vi "Read FP Control.vi"(6 "Field name":string, 8 "error in (no error)":errorcluster, 10 "Control Name":string="Configuration", 11 "Measure Object in":refnum<class "Template Module.lvclass">) -> (0 "error out":errorcluster, 1 "Present":bool, 2 "Control Value":variant, 3 "Measure Object out":refnum<class "Template Module.lvclass">)   [LabVIEW 2018, in "Template Module.lvclass"]
uses:
  Template Module.lvclass
  Template Module.lvclass/Template Module.ctl
  Read Front Panel ref.vi
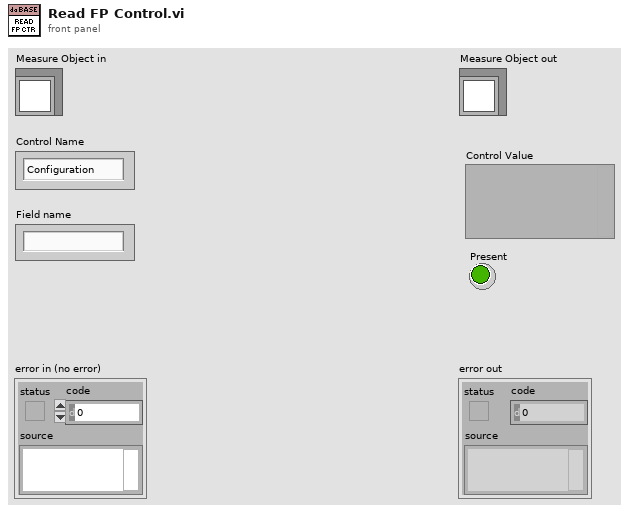
[diagram p1: front panel]
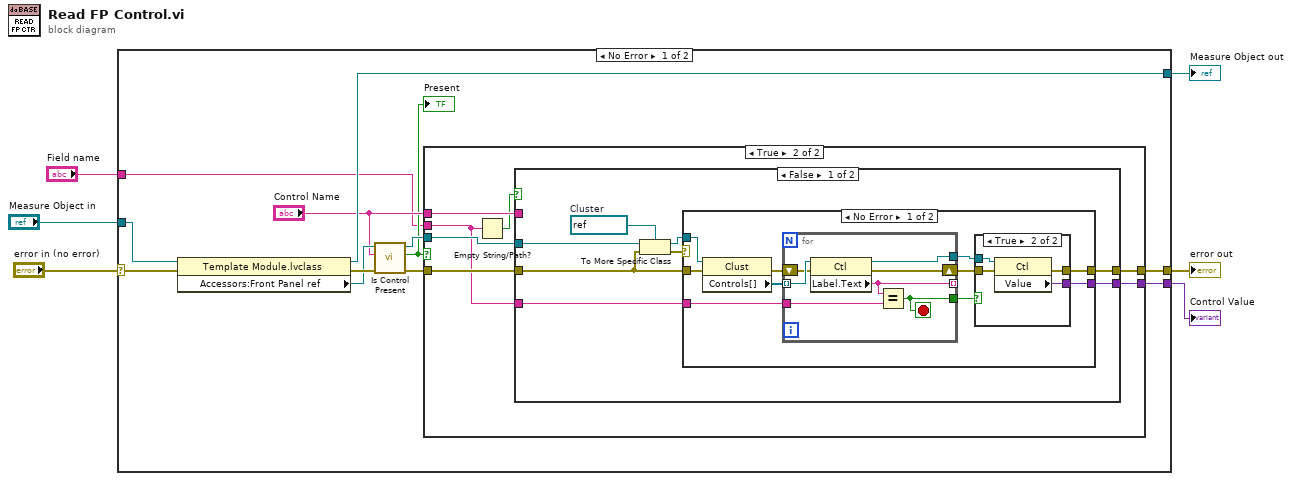
[diagram p0: block diagram]
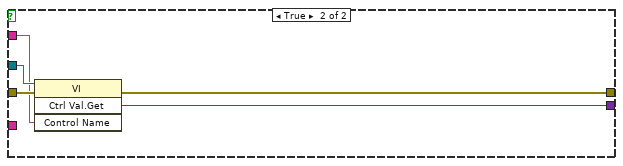
[diagram p5: hidden frame]
diagram:
  n1 = case shown="No Error" "error in (no error)" {
    selector: "error in (no error)" -> [w18 w64]
    tunnel: [w15 w64] -> w5
    tunnel: [w16 w63] -> w3
    tunnel: "Measure Object in" -> [w17 w63]
    tunnel: "Field name" -> [w8 _]
    tunnel: [w7 _] -> w1
    frame No Error {
      n2 = property class="Template Module.lvclass"(reference=w17, error in=w18) -> (reference out=w16:refnum<class "Template Module.lvclass">, error out=w14:errorcluster, "Accessors:Front Panel ref"=w13:refnum<vi>)
      n3 = call "Is Control Present.vi"("Error In"=w14, "Control label"="Control Name", "VI ref"=w13) -> ("Error Out"=w11:errorcluster, "Present"=w9:bool, "VI ref out"=w12:refnum<vi>)  [unwired: 5 in, 1 out]
      "Present" <- w9
      n4 = case shown="True" w9 {
        tunnel: [w19 w26] -> w15
        tunnel: w12 -> [_ w25]
        tunnel: w11 -> [w19 w24]
        tunnel: "Control Name" -> [_ w23]
        tunnel: w8 -> [_ w21]
        tunnel: [_ w20] -> w7
        frame False {
        }
        frame True {
          n5 = Empty String/Path?(string/path=w21) -> (empty?=w22:bool)
          n6 = case shown="False" w22 {
            tunnel: [w27 w62] -> w26
            tunnel: w25 -> [w30 w61]
            tunnel: w24 -> [w29 w60]
            tunnel: w23 -> [_ w59]
            tunnel: w21 -> [w31 _]
            tunnel: [w28 w58] -> w20
            frame False {
              w32 = refnum<vi> refnum  # Cluster
              n7 = To More Specific Class(target class=w32, reference=w30, error in=w29) -> (specific class reference=w34:refnum<vi>, error out=w33:errorcluster)
              n8 = case shown="No Error" w33 {
                tunnel: w34 -> [w43 _]
                tunnel: w29 -> [w42 w57]
                tunnel: w31 -> [w40 _]
                tunnel: [w36 w57] -> w27
                tunnel: [w35 _] -> w28
                frame No Error {
                  n9 = property class="Clust"(reference=w43, error in=w42) -> (error out=w41:errorcluster, "Controls[]"=w44:refnum<vi>[])  [unwired: 1 out]
                  n10 = for {
                    tunnel: w44 -> [w56] mode=indexing
                    tunnel: [w53] -> _ mode=indexing
                    shift-right: [w54] -> w37
                    shift-left: w41 -> [w55]
                    tunnel: w40 -> [w52]
                    tunnel: [w51] -> w38
                    tunnel: [w50] -> w39
                    stop <- w50 stop-if-true
                    n11 = property class="Ctl"(reference=w56, error in=w55) -> (reference out=w51:refnum<vi>, error out=w54:errorcluster, "Label.Text"=w53:string)
                    n12 = Equal?(x=w53, y=w52) -> (x = y?=w50:bool)
                  }
                  n13 = case shown="True" w39 {
                    tunnel: w38 -> [_ w49]
                    tunnel: w37 -> [w45 w48]
                    tunnel: [w45 w47] -> w36
                    tunnel: [_ w46] -> w35
                    frame False {
                    }
                    frame True {
                      n14 = property class="Ctl"(reference=w49, error in=w48) -> (error out=w47:errorcluster, "Value"=w46:variant)  [unwired: 1 out]
                    }
                  }
                }
                frame Error {
                }
              }
            }
            frame True {
              n15 = invoke class="VI" method="Ctrl Val.Get"(reference=w61, error in=w60, "Control Name"=w59) -> (error out=w62:errorcluster, "Get Control Value Variant"=w58:variant)  [unwired: 1 in, 2 out]
            }
          }
        }
      }
    }
    frame Error {
    }
  }
  "error out" <- w5
  "Measure Object out" <- w3
  "Control Value" <- w1
